vi "testDBMec.vi"() -> ()   [LabVIEW 2014]
panel:
  in  "FinMedicion":bool caption="Fin Medicion de Varillas?"
  in  "CreoEnDBTuplaTablaImagen":bool caption="Creo DB Tupla Imagen"
  in  "CreoEnDBTuplaTablaProductoAfterTuplaTablaReceta":bool caption="Insertar Tupla En DB Producto"
  in  "stop":bool
  in  "EstadoActual":string caption="Estado Actual de la Secuencia"
  in  "FinGuardadoMedicion":bool caption="Fin Del Guardado Medicion"
  in  "CreoDBTuplaVarilla":bool caption="Creo DB Tupla Varilla"
  in  "CreoMemorNuevoObjetoImagen":bool caption="Creo Memoria Nuevo Objeto Imagen"
  in  "CreoMemoriaNuevoObjetoRod":bool caption="Creo Memoria Nuevo Objeto Rod"
  in  "CreoEnDBTuplaTablaReceta":bool caption="Inserto Tupla Tabla Receta"
  in  "CreoObjetoRecetaNuevaODSteelGrade":bool caption="Creo Objeto Receta Nueva Para OD SG"
  in  "FinCreacionTuplasDB":bool caption="Fin Creacion Tuplas en DB Producto"
  in  "CreoTuplaEnDBProducto":bool caption="Insertar Tupla En DB Producto"
  in  "SeleccionarReceta":bool caption="Seleccionar Receta De Lista Mostrada"
  in  "MostrarListaRecetas":bool caption="Mostrar Lista de Recetas Existentes OD y SteelGrade"
  in  "VerificarExisteRecetaParaODYSteelGrade":bool caption="Verificar Existe Receta Para OD Y SteelGrade?"
  in  "CrearNuevoObjetoProducto":bool caption="Crear Nuevo Objeto Producto"
  in  "VerificarExisteProducto":bool caption="Verificar  Existe Producto?"
  in  "IngresarODSteelGradeLote":bool caption="Ingresar OD SteelGrade Lote"
  in  "RealizarMedicion":bool caption="Realizar Medicion"
  in  "NewProduct":bool caption="Nuevo Producto?"
  in  "Inicio":bool
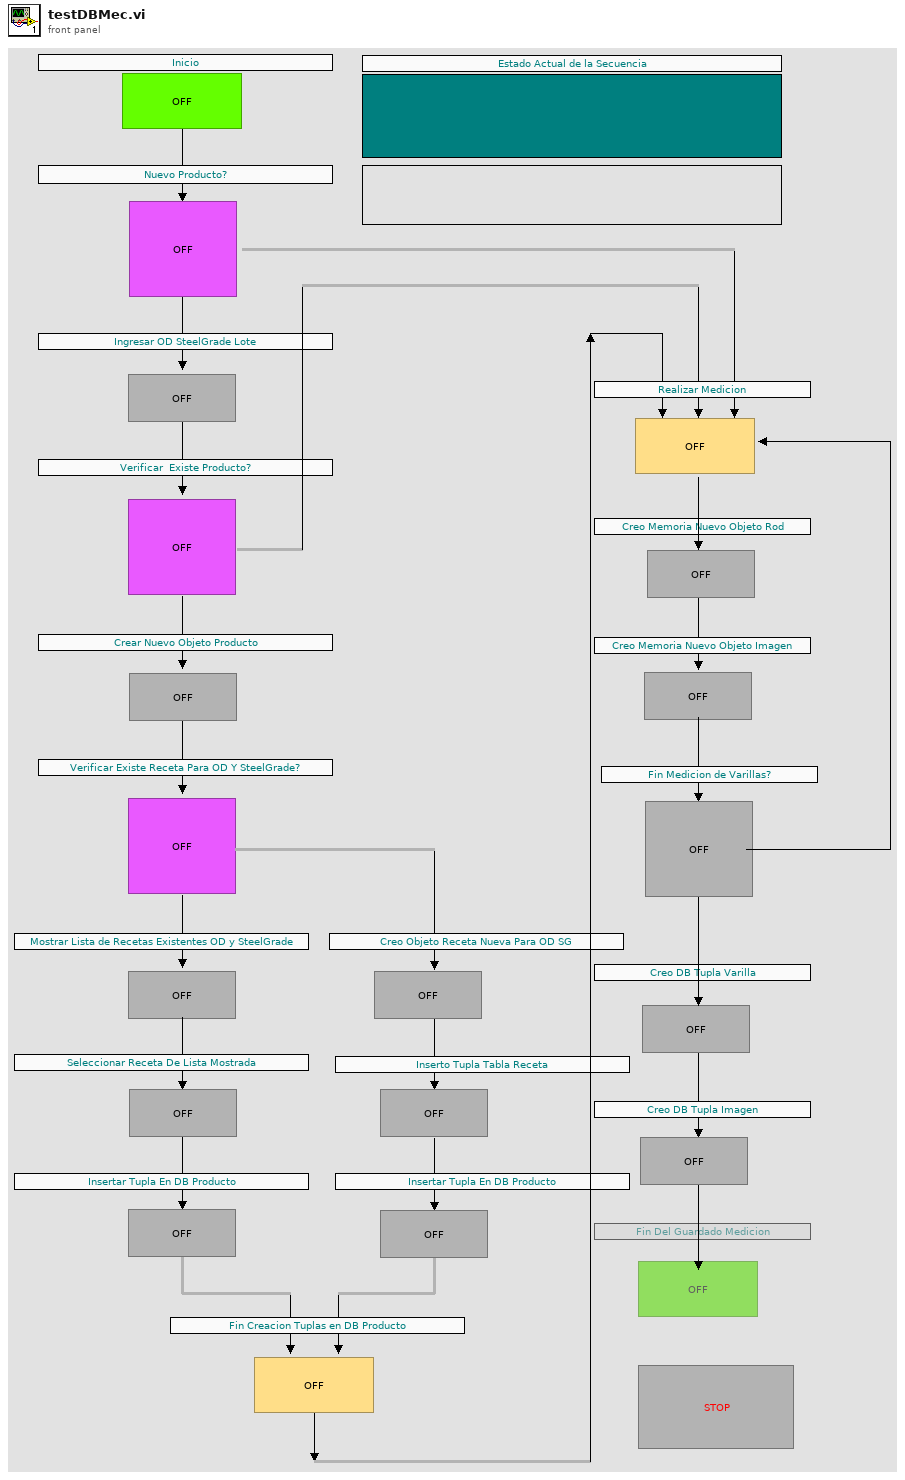
[diagram p1: front panel]
types:
  T1 = enum8{"Enabled", "Disabled", "Disabled and Grayed Out"}
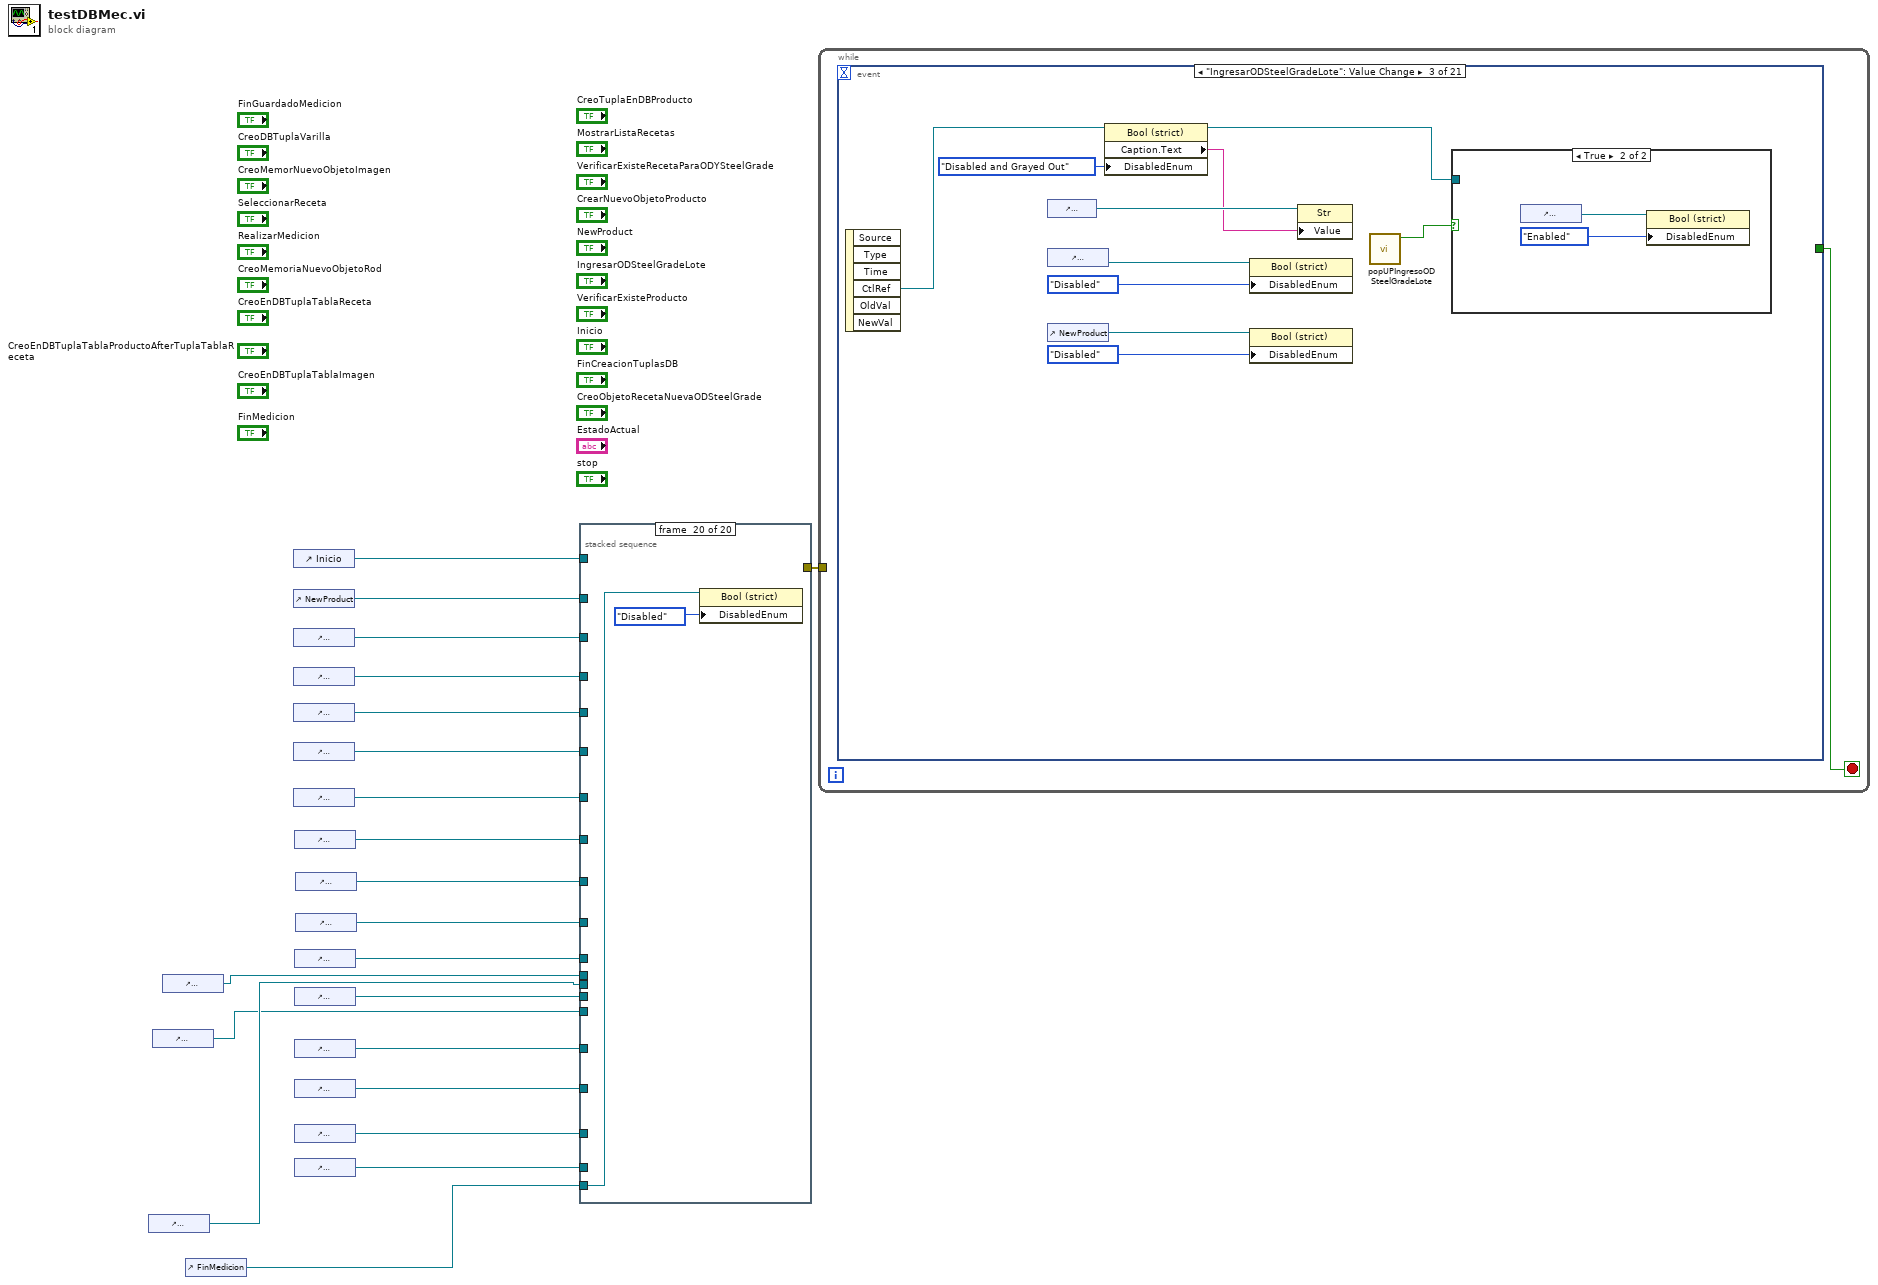
[diagram p0: block diagram]
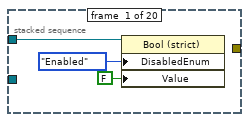
[diagram p2: hidden frame]
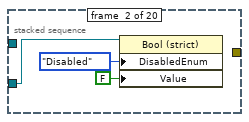
[diagram p3: hidden frame]
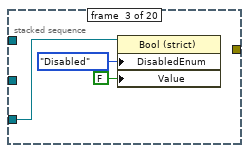
[diagram p4: hidden frame]
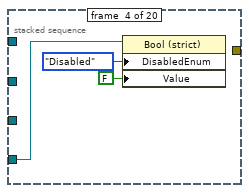
[diagram p5: hidden frame]
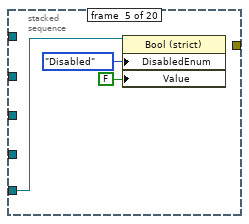
[diagram p6: hidden frame]
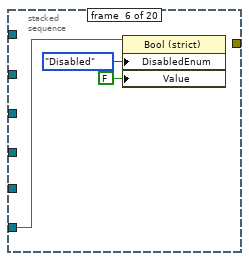
[diagram p7: hidden frame]
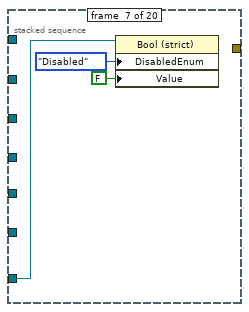
[diagram p8: hidden frame]
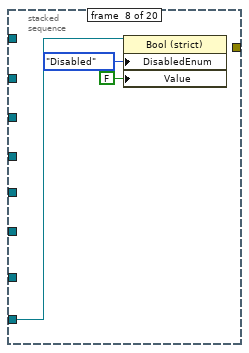
[diagram p9: hidden frame]
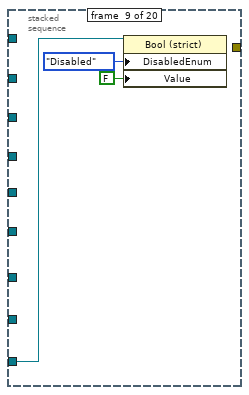
[diagram p10: hidden frame]
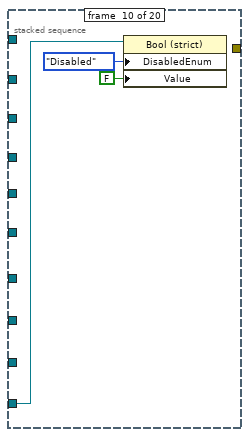
[diagram p11: hidden frame]
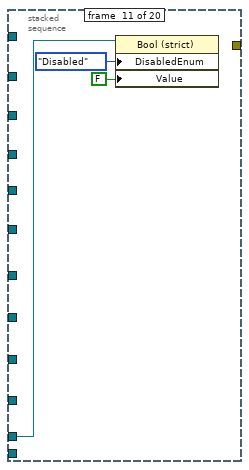
[diagram p12: hidden frame]
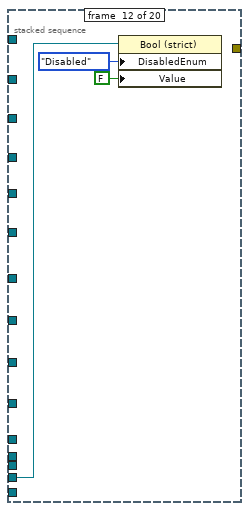
[diagram p13: hidden frame]
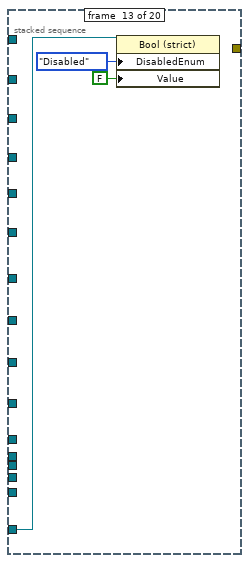
[diagram p14: hidden frame]
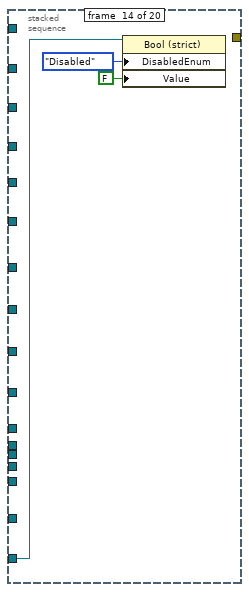
[diagram p15: hidden frame]
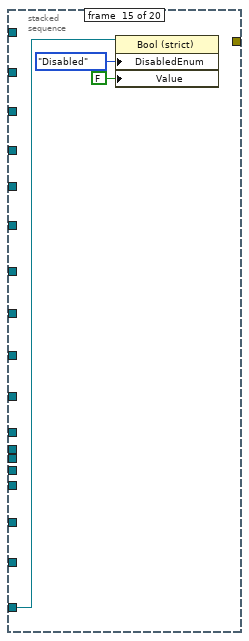
[diagram p16: hidden frame]
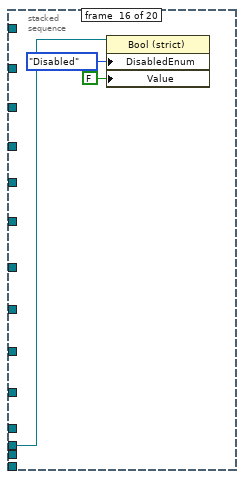
[diagram p17: hidden frame]
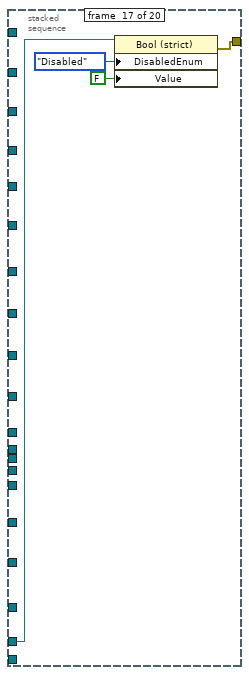
[diagram p18: hidden frame]
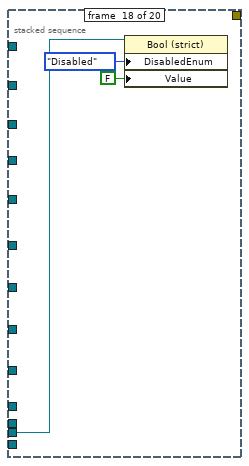
[diagram p19: hidden frame]
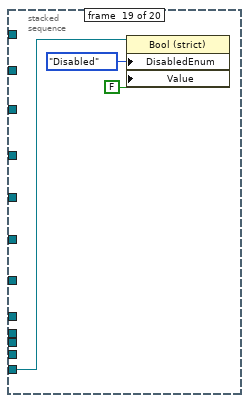
[diagram p20: hidden frame]
diagram:
  n1 = control-ref of="CreoEnDBTuplaTablaProductoAfterTuplaTablaReceta"() -> (w3:refnum<vi>)
  n2 = control-ref of="CreoEnDBTuplaTablaImagen"() -> (w2:refnum<vi>)
  n3 = control-ref of="FinCreacionTuplasDB"() -> (w4:refnum<vi>)
  n4 = control-ref of="FinMedicion"() -> (w1:refnum<vi>)
  n5 = control-ref of="Inicio"() -> (w21:refnum<vi>)
  n6 = control-ref of="NewProduct"() -> (w20:refnum<vi>)
  n7 = control-ref of="IngresarODSteelGradeLote"() -> (w19:refnum<vi>)
  n8 = control-ref of="VerificarExisteProducto"() -> (w18:refnum<vi>)
  n9 = control-ref of="CrearNuevoObjetoProducto"() -> (w17:refnum<vi>)
  n10 = control-ref of="VerificarExisteRecetaParaODYSteelGrade"() -> (w16:refnum<vi>)
  n11 = control-ref of="MostrarListaRecetas"() -> (w15:refnum<vi>)
  n12 = control-ref of="SeleccionarReceta"() -> (w14:refnum<vi>)
  n13 = control-ref of="CreoEnDBTuplaTablaReceta"() -> (w11:refnum<vi>)
  n14 = control-ref of="RealizarMedicion"() -> (w9:refnum<vi>)
  n15 = control-ref of="CreoMemoriaNuevoObjetoRod"() -> (w8:refnum<vi>)
  n16 = control-ref of="CreoMemorNuevoObjetoImagen"() -> (w7:refnum<vi>)
  n17 = control-ref of="CreoDBTuplaVarilla"() -> (w6:refnum<vi>)
  n18 = control-ref of="FinGuardadoMedicion"() -> (w5:refnum<vi>)
  n19 = control-ref of="CreoTuplaEnDBProducto"() -> (w13:refnum<vi>)
  n20 = control-ref of="CreoObjetoRecetaNuevaODSteelGrade"() -> (w12:refnum<vi>)
  n21 = stacked-sequence {
    tunnel: w21 -> [w24 _ _ _ _ _ _ _ _ _ _ _ _ _ _ _ _ _ _ _]
    tunnel: w20 -> [_ w27 _ _ _ _ _ _ _ _ _ _ _ _ _ _ _ _ _ _]
    tunnel: w19 -> [_ _ w30 _ _ _ _ _ _ _ _ _ _ _ _ _ _ _ _ _]
    tunnel: w18 -> [_ _ _ w33 _ _ _ _ _ _ _ _ _ _ _ _ _ _ _ _]
    tunnel: w17 -> [_ _ _ _ w36 _ _ _ _ _ _ _ _ _ _ _ _ _ _ _]
    tunnel: w16 -> [_ _ _ _ _ w39 _ _ _ _ _ _ _ _ _ _ _ _ _ _]
    tunnel: w15 -> [_ _ _ _ _ _ w42 _ _ _ _ _ _ _ _ _ _ _ _ _]
    tunnel: w14 -> [_ _ _ _ _ _ _ w45 _ _ _ _ _ _ _ _ _ _ _ _]
    tunnel: w13 -> [_ _ _ _ _ _ _ _ w48 _ _ _ _ _ _ _ _ _ _ _]
    tunnel: w12 -> [_ _ _ _ _ _ _ _ _ w51 _ _ _ _ _ _ _ _ _ _]
    tunnel: w11 -> [_ _ _ _ _ _ _ _ _ _ w54 _ _ _ _ _ _ _ _ _]
    tunnel: [_ _ _ _ _ _ _ _ _ _ _ _ _ _ _ _ w71 _ _ _] -> w10
    tunnel: w9 -> [_ _ _ _ _ _ _ _ _ _ _ w57 _ _ _ _ _ _ _ _]
    tunnel: w8 -> [_ _ _ _ _ _ _ _ _ _ _ _ w60 _ _ _ _ _ _ _]
    tunnel: w7 -> [_ _ _ _ _ _ _ _ _ _ _ _ _ w63 _ _ _ _ _ _]
    tunnel: w6 -> [_ _ _ _ _ _ _ _ _ _ _ _ _ _ w66 _ _ _ _ _]
    tunnel: w5 -> [_ _ _ _ _ _ _ _ _ _ _ _ _ _ _ _ w73 _ _ _]
    tunnel: w4 -> [_ _ _ _ _ _ _ _ _ _ _ _ _ _ _ w69 _ _ _ _]
    tunnel: w3 -> [_ _ _ _ _ _ _ _ _ _ _ _ _ _ _ _ _ w76 _ _]
    tunnel: w2 -> [_ _ _ _ _ _ _ _ _ _ _ _ _ _ _ _ _ _ w79 _]
    tunnel: w1 -> [_ _ _ _ _ _ _ _ _ _ _ _ _ _ _ _ _ _ _ w81]
    frame #0 {
      n22 = property class="Bool (strict)"(reference=w24, "DisabledEnum"=T1."Enabled" ("Disabled"), "Value"=FALSE) -> ()  [unwired: 1 in, 2 out]
    }
    frame #1 {
      n23 = property class="Bool (strict)"(reference=w27, "DisabledEnum"=T1."Disabled" ("Disabled"), "Value"=FALSE) -> ()  [unwired: 1 in, 2 out]
    }
    frame #2 {
      n24 = property class="Bool (strict)"(reference=w30, "DisabledEnum"=T1."Disabled" ("Disabled"), "Value"=FALSE) -> ()  [unwired: 1 in, 2 out]
    }
    frame #3 {
      n25 = property class="Bool (strict)"(reference=w33, "DisabledEnum"=T1."Disabled" ("Disabled"), "Value"=FALSE) -> ()  [unwired: 1 in, 2 out]
    }
    frame #4 {
      n26 = property class="Bool (strict)"(reference=w36, "DisabledEnum"=T1."Disabled" ("Disabled"), "Value"=FALSE) -> ()  [unwired: 1 in, 2 out]
    }
    frame #5 {
      n27 = property class="Bool (strict)"(reference=w39, "DisabledEnum"=T1."Disabled" ("Disabled"), "Value"=FALSE) -> ()  [unwired: 1 in, 2 out]
    }
    frame #6 {
      n28 = property class="Bool (strict)"(reference=w42, "DisabledEnum"=T1."Disabled" ("Disabled"), "Value"=FALSE) -> ()  [unwired: 1 in, 2 out]
    }
    frame #7 {
      n29 = property class="Bool (strict)"(reference=w45, "DisabledEnum"=T1."Disabled" ("Disabled"), "Value"=FALSE) -> ()  [unwired: 1 in, 2 out]
    }
    frame #8 {
      n30 = property class="Bool (strict)"(reference=w48, "DisabledEnum"=T1."Disabled" ("Disabled"), "Value"=FALSE) -> ()  [unwired: 1 in, 2 out]
    }
    frame #9 {
      n31 = property class="Bool (strict)"(reference=w51, "DisabledEnum"=T1."Disabled" ("Disabled"), "Value"=FALSE) -> ()  [unwired: 1 in, 2 out]
    }
    frame #10 {
      n32 = property class="Bool (strict)"(reference=w54, "DisabledEnum"=T1."Disabled" ("Disabled"), "Value"=FALSE) -> ()  [unwired: 1 in, 2 out]
    }
    frame #11 {
      n33 = property class="Bool (strict)"(reference=w57, "DisabledEnum"=T1."Disabled" ("Disabled"), "Value"=FALSE) -> ()  [unwired: 1 in, 2 out]
    }
    frame #12 {
      n34 = property class="Bool (strict)"(reference=w60, "DisabledEnum"=T1."Disabled" ("Disabled"), "Value"=FALSE) -> ()  [unwired: 1 in, 2 out]
    }
    frame #13 {
      n35 = property class="Bool (strict)"(reference=w63, "DisabledEnum"=T1."Disabled" ("Disabled"), "Value"=FALSE) -> ()  [unwired: 1 in, 2 out]
    }
    frame #14 {
      n36 = property class="Bool (strict)"(reference=w66, "DisabledEnum"=T1."Disabled" ("Disabled"), "Value"=FALSE) -> ()  [unwired: 1 in, 2 out]
    }
    frame #15 {
      n37 = property class="Bool (strict)"(reference=w69, "DisabledEnum"=T1."Disabled" ("Disabled"), "Value"=FALSE) -> ()  [unwired: 1 in, 2 out]
    }
    frame #16 {
      n38 = property class="Bool (strict)"(reference=w73, "DisabledEnum"=T1."Disabled" ("Disabled"), "Value"=FALSE) -> (error out=w71:errorcluster)  [unwired: 1 in, 1 out]
    }
    frame #17 {
      n39 = property class="Bool (strict)"(reference=w76, "DisabledEnum"=T1."Disabled" ("Disabled"), "Value"=FALSE) -> ()  [unwired: 1 in, 2 out]
    }
    frame #18 {
      n40 = property class="Bool (strict)"(reference=w79, "DisabledEnum"=T1."Disabled" ("Disabled"), "Value"=FALSE) -> ()  [unwired: 1 in, 2 out]
    }
    frame #19 {
      n41 = property class="Bool (strict)"(reference=w81, "DisabledEnum"=T1."Disabled" ("Disabled")) -> ()  [unwired: 1 in, 2 out]
    }
  }
  n42 = while {
    tunnel: w10 -> [_]
    stop <- w82 stop-if-true
    n43 = event shown="[2] \"IngresarODSteelGradeLote\": Value Change" {
      selector: _ -> [_ _ _ _ _ _ _ _ _ _ _ _ _ _ _ _ _ _ _ _ _]
      dyn-events: _ -> [_ _ _ _ _ _ _ _ _ _ _ _ _ _ _ _ _ _ _ _ _]
      timeout: _ -> [_ _ _ _ _ _ _ _ _ _ _ _ _ _ _ _ _ _ _ _ _]
      tunnel: [_ _ _ _ _ _ _ _ _ _ _ _ _ _ _ _ _ _ _ _ w355] -> w82
      event "Inicio": Value Change {
        n44 = event-data() -> ("CtlRef"=w88:refnum<vi>)  [unwired: 1 in, 5 out]
        n45 = control-ref of="EstadoActual"() -> (w87:refnum<vi>)
        n46 = control-ref of="NewProduct"() -> (w85:refnum<vi>)
        n47 = property class="Bool (strict)"(reference=w88, "DisabledEnum"=T1."Disabled and Grayed Out" ("Disabled")) -> ("Caption.Text"=w86:string)  [unwired: 1 in, 2 out]
        n48 = property class="Bool (strict)"(reference=w85, "DisabledEnum"=T1."Enabled" ("Disabled")) -> ()  [unwired: 1 in, 2 out]
        n49 = property class="Str"(reference=w87, "Value"=w86) -> ()  [unwired: 1 in, 2 out]
      }
      event "NewProduct": Value Change {
        n50 = event-data() -> ("CtlRef"=w95:refnum<vi>)  [unwired: 1 in, 5 out]
        n51 = control-ref of="EstadoActual"() -> (w94:refnum<vi>)
        n52 = control-ref of="Inicio"() -> (w92:refnum<vi>)
        n53 = property class="Bool (strict)"(reference=w95, "DisabledEnum"=T1."Disabled and Grayed Out" ("Disabled")) -> ("Caption.Text"=w93:string)  [unwired: 1 in, 2 out]
        n54 = property class="Bool (strict)"(reference=w92, "DisabledEnum"=T1."Disabled" ("Disabled")) -> ()  [unwired: 1 in, 2 out]
        n55 = property class="Str"(reference=w94, "Value"=w93) -> ()  [unwired: 1 in, 2 out]
        n56 = call "popUPSINO.vi"() -> ("estadoConsulta"=w89:bool)  [unwired: 11 in]
        n57 = case shown="False" w89 {
          frame False {
            n58 = control-ref of="RealizarMedicion"() -> (w96:refnum<vi>)
            n59 = property class="Bool (strict)"(reference=w96, "DisabledEnum"=T1."Enabled" ("Disabled")) -> ()  [unwired: 1 in, 2 out]
          }
          frame True {
            n60 = control-ref of="IngresarODSteelGradeLote"() -> (w99:refnum<vi>)
            n61 = property class="Bool (strict)"(reference=w99, "DisabledEnum"=T1."Enabled" ("Disabled")) -> ()  [unwired: 1 in, 2 out]
          }
        }
      }
      event "IngresarODSteelGradeLote": Value Change {
        n62 = event-data() -> ("CtlRef"=w109:refnum<vi>)  [unwired: 1 in, 5 out]
        n63 = control-ref of="EstadoActual"() -> (w108:refnum<vi>)
        n64 = control-ref of="RealizarMedicion"() -> (w104:refnum<vi>)
        n65 = control-ref of="NewProduct"() -> (w106:refnum<vi>)
        n66 = property class="Bool (strict)"(reference=w109, "DisabledEnum"=T1."Disabled and Grayed Out" ("Disabled")) -> (reference out=w101:refnum<vi>, "Caption.Text"=w107:string)  [unwired: 1 in, 1 out]
        n67 = property class="Bool (strict)"(reference=w104, "DisabledEnum"=T1."Disabled" ("Disabled")) -> ()  [unwired: 1 in, 2 out]
        n68 = property class="Bool (strict)"(reference=w106, "DisabledEnum"=T1."Disabled" ("Disabled")) -> ()  [unwired: 1 in, 2 out]
        n69 = property class="Str"(reference=w108, "Value"=w107) -> ()  [unwired: 1 in, 2 out]
        n70 = call "popUPIngresoODSteelGradeLote.vi"() -> ("Listo Ingresar OD SteelGrade Lote"=w100:bool)  [unwired: 10 in, 1 out]
        n71 = case shown="True" w100 {
          tunnel: w101 -> [_ _]
          frame False {
          }
          frame True {
            n72 = control-ref of="VerificarExisteProducto"() -> (w111:refnum<vi>)
            n73 = property class="Bool (strict)"(reference=w111, "DisabledEnum"=T1."Enabled" ("Disabled")) -> ()  [unwired: 1 in, 2 out]
          }
        }
      }
      event "VerificarExisteProducto": Value Change {
        n74 = event-data() -> ("CtlRef"=w118:refnum<vi>)  [unwired: 1 in, 5 out]
        n75 = control-ref of="EstadoActual"() -> (w117:refnum<vi>)
        n76 = control-ref of="IngresarODSteelGradeLote"() -> (w115:refnum<vi>)
        n77 = property class="Bool (strict)"(reference=w118, "DisabledEnum"=T1."Disabled and Grayed Out" ("Disabled")) -> ("Caption.Text"=w116:string)  [unwired: 1 in, 2 out]
        n78 = property class="Bool (strict)"(reference=w115, "DisabledEnum"=T1."Disabled" ("Disabled")) -> ()  [unwired: 1 in, 2 out]
        n79 = property class="Str"(reference=w117, "Value"=w116) -> ()  [unwired: 1 in, 2 out]
        n80 = call "popUPSINO.vi"() -> ("estadoConsulta"=w112:bool)  [unwired: 11 in]
        n81 = case shown="False" w112 {
          frame False {
            n82 = control-ref of="CrearNuevoObjetoProducto"() -> (w119:refnum<vi>)
            n83 = property class="Bool (strict)"(reference=w119, "DisabledEnum"=T1."Enabled" ("Disabled")) -> ()  [unwired: 1 in, 2 out]
          }
          frame True {
            n84 = control-ref of="RealizarMedicion"() -> (w121:refnum<vi>)
            n85 = property class="Bool (strict)"(reference=w121, "DisabledEnum"=T1."Enabled" ("Disabled")) -> ()  [unwired: 1 in, 2 out]
          }
        }
      }
      event "CrearNuevoObjetoProducto": Value Change {
        n86 = event-data() -> ("CtlRef"=w131:refnum<vi>)  [unwired: 1 in, 5 out]
        n87 = control-ref of="EstadoActual"() -> (w130:refnum<vi>)
        n88 = control-ref of="VerificarExisteProducto"() -> (w129:refnum<vi>)
        n89 = control-ref of="RealizarMedicion"() -> (w127:refnum<vi>)
        n90 = property class="Bool (strict)"(reference=w131, "DisabledEnum"=T1."Disabled and Grayed Out" ("Disabled")) -> ("Caption.Text"=w124:string)  [unwired: 1 in, 2 out]
        n91 = property class="Bool (strict)"(reference=w129, "DisabledEnum"=T1."Disabled" ("Disabled")) -> ()  [unwired: 1 in, 2 out]
        n92 = property class="Bool (strict)"(reference=w127, "DisabledEnum"=T1."Disabled" ("Disabled")) -> ()  [unwired: 1 in, 2 out]
        n93 = property class="Str"(reference=w130, "Value"=w124) -> ()  [unwired: 1 in, 2 out]
        n94 = call "popUPCrearNuevoObjetoProducto.vi"() -> ("Listo Ingresar objeto Producto"=w123:bool)  [unwired: 11 in]
        n95 = case shown="True" w123 {
          frame False {
          }
          frame True {
            n96 = control-ref of="VerificarExisteRecetaParaODYSteelGrade"() -> (w132:refnum<vi>)
            n97 = property class="Bool (strict)"(reference=w132, "DisabledEnum"=T1."Enabled" ("Disabled")) -> ()  [unwired: 1 in, 2 out]
          }
        }
      }
      event "VerificarExisteRecetaParaODYSteelGrade": Value Change {
        n98 = event-data() -> ("CtlRef"=w140:refnum<vi>)  [unwired: 1 in, 5 out]
        n99 = control-ref of="EstadoActual"() -> (w139:refnum<vi>)
        n100 = control-ref of="CrearNuevoObjetoProducto"() -> (w137:refnum<vi>)
        n101 = property class="Bool (strict)"(reference=w140, "DisabledEnum"=T1."Disabled and Grayed Out" ("Disabled")) -> ("Caption.Text"=w138:string)  [unwired: 1 in, 2 out]
        n102 = property class="Bool (strict)"(reference=w137, "DisabledEnum"=T1."Disabled" ("Disabled")) -> ()  [unwired: 1 in, 2 out]
        n103 = property class="Str"(reference=w139, "Value"=w138) -> ()  [unwired: 1 in, 2 out]
        n104 = call "popUPSINO.vi"() -> ("estadoConsulta"=w134:bool)  [unwired: 11 in]
        n105 = case shown="False" w134 {
          frame False {
            n106 = control-ref of="CreoObjetoRecetaNuevaODSteelGrade"() -> (w141:refnum<vi>)
            n107 = property class="Bool (strict)"(reference=w141, "DisabledEnum"=T1."Enabled" ("Disabled")) -> ()  [unwired: 1 in, 2 out]
          }
          frame True {
            n108 = control-ref of="MostrarListaRecetas"() -> (w143:refnum<vi>)
            n109 = property class="Bool (strict)"(reference=w143, "DisabledEnum"=T1."Enabled" ("Disabled")) -> ()  [unwired: 1 in, 2 out]
          }
        }
      }
      event "MostrarListaRecetas": Value Change {
        n110 = event-data() -> ("CtlRef"=w153:refnum<vi>)  [unwired: 1 in, 5 out]
        n111 = control-ref of="EstadoActual"() -> (w152:refnum<vi>)
        n112 = control-ref of="VerificarExisteRecetaParaODYSteelGrade"() -> (w150:refnum<vi>)
        n113 = control-ref of="CreoObjetoRecetaNuevaODSteelGrade"() -> (w148:refnum<vi>)
        n114 = property class="Bool (strict)"(reference=w153, "DisabledEnum"=T1."Disabled and Grayed Out" ("Disabled")) -> ("Caption.Text"=w151:string)  [unwired: 1 in, 2 out]
        n115 = property class="Bool (strict)"(reference=w150, "DisabledEnum"=T1."Disabled" ("Disabled")) -> ()  [unwired: 1 in, 2 out]
        n116 = property class="Bool (strict)"(reference=w148, "DisabledEnum"=T1."Disabled" ("Disabled")) -> ()  [unwired: 1 in, 2 out]
        n117 = property class="Str"(reference=w152, "Value"=w151) -> ()  [unwired: 1 in, 2 out]
        n118 = call "popUPConsultaListaRecetas.vi"() -> ("Listo ListarRecetas"=w145:bool)  [unwired: 11 in]
        n119 = case shown="True" w145 {
          frame False {
          }
          frame True {
            n120 = control-ref of="SeleccionarReceta"() -> (w154:refnum<vi>)
            n121 = property class="Bool (strict)"(reference=w154, "DisabledEnum"=T1."Enabled" ("Disabled")) -> ()  [unwired: 1 in, 2 out]
          }
        }
      }
      event "SeleccionarReceta": Value Change {
        n122 = event-data() -> ("CtlRef"=w164:refnum<vi>)  [unwired: 1 in, 5 out]
        n123 = control-ref of="EstadoActual"() -> (w163:refnum<vi>)
        n124 = control-ref of="MostrarListaRecetas"() -> (w161:refnum<vi>)
        n125 = property class="Bool (strict)"(reference=w164, "DisabledEnum"=T1."Disabled and Grayed Out" ("Disabled")) -> ("Caption.Text"=w162:string)  [unwired: 1 in, 2 out]
        n126 = property class="Bool (strict)"(reference=w161, "DisabledEnum"=T1."Disabled" ("Disabled")) -> ()  [unwired: 1 in, 2 out]
        n127 = property class="Str"(reference=w163, "Value"=w162) -> ()  [unwired: 1 in, 2 out]
        n128 = call "popUPSeleccionReceta.vi"() -> ("idReceta"=w156:string, "recetaSeleccionadaDeLaLista"=w157:string, "Listo SeleccionListaDeReceta"=w158:bool)  [unwired: 9 in]
        n129 = case shown="True" w158 {
          tunnel: w157 -> [_ _]
          tunnel: w156 -> [_ _]
          frame False {
          }
          frame True {
            n130 = control-ref of="CreoTuplaEnDBProducto"() -> (w165:refnum<vi>)
            n131 = property class="Bool (strict)"(reference=w165, "DisabledEnum"=T1."Enabled" ("Disabled")) -> ()  [unwired: 1 in, 2 out]
          }
        }
      }
      event "CreoTuplaEnDBProducto": Value Change {
        n132 = event-data() -> ("CtlRef"=w173:refnum<vi>)  [unwired: 1 in, 5 out]
        n133 = control-ref of="EstadoActual"() -> (w172:refnum<vi>)
        n134 = control-ref of="SeleccionarReceta"() -> (w170:refnum<vi>)
        n135 = property class="Bool (strict)"(reference=w173, "DisabledEnum"=T1."Disabled and Grayed Out" ("Disabled")) -> ("Caption.Text"=w171:string)  [unwired: 1 in, 2 out]
        n136 = property class="Bool (strict)"(reference=w170, "DisabledEnum"=T1."Disabled" ("Disabled")) -> ()  [unwired: 1 in, 2 out]
        n137 = property class="Str"(reference=w172, "Value"=w171) -> ()  [unwired: 1 in, 2 out]
        n138 = call "popUPInsertarTuplaEnDBProducto.vi"() -> ("ListoGuardarEnDB"=w167:bool)  [unwired: 11 in]
        n139 = case shown="True" w167 {
          frame False {
          }
          frame True {
            n140 = control-ref of="FinCreacionTuplasDB"() -> (w174:refnum<vi>)
            n141 = property class="Bool (strict)"(reference=w174, "DisabledEnum"=T1."Enabled" ("Disabled")) -> ()  [unwired: 1 in, 2 out]
          }
        }
      }
      event "CreoObjetoRecetaNuevaODSteelGrade": Value Change {
        n142 = event-data() -> ("CtlRef"=w184:refnum<vi>)  [unwired: 1 in, 5 out]
        n143 = control-ref of="EstadoActual"() -> (w183:refnum<vi>)
        n144 = control-ref of="VerificarExisteRecetaParaODYSteelGrade"() -> (w181:refnum<vi>)
        n145 = control-ref of="MostrarListaRecetas"() -> (w179:refnum<vi>)
        n146 = property class="Bool (strict)"(reference=w184, "DisabledEnum"=T1."Disabled and Grayed Out" ("Disabled")) -> ("Caption.Text"=w182:string)  [unwired: 1 in, 2 out]
        n147 = property class="Bool (strict)"(reference=w181, "DisabledEnum"=T1."Disabled" ("Disabled")) -> ()  [unwired: 1 in, 2 out]
        n148 = property class="Bool (strict)"(reference=w179, "DisabledEnum"=T1."Disabled" ("Disabled")) -> ()  [unwired: 1 in, 2 out]
        n149 = property class="Str"(reference=w183, "Value"=w182) -> ()  [unwired: 1 in, 2 out]
        n150 = call "popUPCrearNuevoObjetoReceta.vi"() -> ("Listo Ingresar OD SteelGrade Lote"=w176:bool)  [unwired: 10 in, 1 out]
        n151 = case shown="True" w176 {
          frame False {
          }
          frame True {
            n152 = control-ref of="CreoEnDBTuplaTablaReceta"() -> (w185:refnum<vi>)
            n153 = property class="Bool (strict)"(reference=w185, "DisabledEnum"=T1."Enabled" ("Disabled")) -> ()  [unwired: 1 in, 2 out]
          }
        }
      }
      event "CreoEnDBTuplaTablaReceta": Value Change {
        n154 = event-data() -> ("CtlRef"=w193:refnum<vi>)  [unwired: 1 in, 5 out]
        n155 = property class="Bool (strict)"(reference=w193, "DisabledEnum"=T1."Disabled and Grayed Out" ("Disabled")) -> ("Caption.Text"=w191:string)  [unwired: 1 in, 2 out]
        n156 = control-ref of="EstadoActual"() -> (w192:refnum<vi>)
        n157 = control-ref of="CreoObjetoRecetaNuevaODSteelGrade"() -> (w190:refnum<vi>)
        n158 = property class="Bool (strict)"(reference=w190, "DisabledEnum"=T1."Disabled" ("Disabled")) -> ()  [unwired: 1 in, 2 out]
        n159 = property class="Str"(reference=w192, "Value"=w191) -> ()  [unwired: 1 in, 2 out]
        n160 = call "popUPInsertarTuplaEnDBReceta.vi"() -> ("Listo Ingresar OD SteelGrade Lote"=w187:bool)  [unwired: 11 in]
        n161 = case shown="True" w187 {
          frame False {
          }
          frame True {
            n162 = control-ref of="CreoEnDBTuplaTablaProductoAfterTuplaTablaReceta"() -> (w194:refnum<vi>)
            n163 = property class="Bool (strict)"(reference=w194, "DisabledEnum"=T1."Enabled" ("Disabled")) -> ()  [unwired: 1 in, 2 out]
          }
        }
      }
      event "CreoEnDBTuplaTablaProductoAfterTuplaTablaReceta": Value Change {
        n164 = event-data() -> ("CtlRef"=w202:refnum<vi>)  [unwired: 1 in, 5 out]
        n165 = control-ref of="CreoEnDBTuplaTablaReceta"() -> (w198:refnum<vi>)
        n166 = property class="Bool (strict)"(reference=w202, "DisabledEnum"=T1."Disabled and Grayed Out" ("Disabled")) -> ("Caption.Text"=w199:string)  [unwired: 1 in, 2 out]
        n167 = control-ref of="EstadoActual"() -> (w200:refnum<vi>)
        n168 = property class="Bool (strict)"(reference=w198, "DisabledEnum"=T1."Disabled" ("Disabled")) -> ()  [unwired: 1 in, 2 out]
        n169 = property class="Str"(reference=w200, "Value"=w199) -> ()  [unwired: 1 in, 2 out]
        n170 = call "popUPInsertarTuplaEnDBProducto.vi"() -> ("ListoGuardarEnDB"=w196:bool)  [unwired: 11 in]
        n171 = case shown="True" w196 {
          frame False {
          }
          frame True {
            n172 = control-ref of="FinCreacionTuplasDB"() -> (w204:refnum<vi>)
            n173 = property class="Bool (strict)"(reference=w204, "DisabledEnum"=T1."Enabled" ("Disabled")) -> ()  [unwired: 1 in, 2 out]
          }
        }
      }
      event "FinCreacionTuplasDB": Value Change {
        n174 = event-data() -> ("CtlRef"=w214:refnum<vi>)  [unwired: 1 in, 5 out]
        n175 = control-ref of="EstadoActual"() -> (w213:refnum<vi>)
        n176 = control-ref of="CreoTuplaEnDBProducto"() -> (w211:refnum<vi>)
        n177 = control-ref of="RealizarMedicion"() -> (w208:refnum<vi>)
        n178 = control-ref of="CreoEnDBTuplaTablaProductoAfterTuplaTablaReceta"() -> (w205:refnum<vi>)
        n179 = property class="Bool (strict)"(reference=w214, "DisabledEnum"=T1."Disabled and Grayed Out" ("Disabled")) -> ("Caption.Text"=w212:string)  [unwired: 1 in, 2 out]
        n180 = property class="Bool (strict)"(reference=w211, "DisabledEnum"=T1."Disabled" ("Disabled")) -> ()  [unwired: 1 in, 2 out]
        n181 = property class="Bool (strict)"(reference=w205, "DisabledEnum"=T1."Disabled" ("Disabled")) -> ()  [unwired: 1 in, 2 out]
        n182 = property class="Bool (strict)"(reference=w208, "DisabledEnum"=T1."Enabled" ("Disabled")) -> ()  [unwired: 1 in, 2 out]
        n183 = property class="Str"(reference=w213, "Value"=w212) -> ()  [unwired: 1 in, 2 out]
      }
      event "RealizarMedicion": Value Change {
        n184 = event-data() -> ("CtlRef"=w230:refnum<vi>)  [unwired: 1 in, 5 out]
        n185 = control-ref of="EstadoActual"() -> (w229:refnum<vi>)
        n186 = control-ref of="FinCreacionTuplasDB"() -> (w227:refnum<vi>)
        n187 = control-ref of="VerificarExisteProducto"() -> (w225:refnum<vi>)
        n188 = control-ref of="NewProduct"() -> (w223:refnum<vi>)
        n189 = control-ref of="IngresarODSteelGradeLote"() -> (w219:refnum<vi>)
        n190 = control-ref of="CrearNuevoObjetoProducto"() -> (w217:refnum<vi>)
        n191 = control-ref of="CreoMemoriaNuevoObjetoRod"() -> (w221:refnum<vi>)
        n192 = property class="Bool (strict)"(reference=w230, "DisabledEnum"=T1."Disabled and Grayed Out" ("Disabled")) -> ("Caption.Text"=w228:string)  [unwired: 1 in, 2 out]
        n193 = property class="Bool (strict)"(reference=w227, "DisabledEnum"=T1."Disabled" ("Disabled")) -> ()  [unwired: 1 in, 2 out]
        n194 = property class="Bool (strict)"(reference=w225, "DisabledEnum"=T1."Disabled" ("Disabled")) -> ()  [unwired: 1 in, 2 out]
        n195 = property class="Bool (strict)"(reference=w223, "DisabledEnum"=T1."Disabled" ("Disabled")) -> ()  [unwired: 1 in, 2 out]
        n196 = property class="Bool (strict)"(reference=w219, "DisabledEnum"=T1."Disabled" ("Disabled")) -> ()  [unwired: 1 in, 2 out]
        n197 = property class="Bool (strict)"(reference=w217, "DisabledEnum"=T1."Disabled" ("Disabled")) -> ()  [unwired: 1 in, 2 out]
        n198 = property class="Bool (strict)"(reference=w221, "DisabledEnum"=T1."Enabled" ("Disabled")) -> ()  [unwired: 1 in, 2 out]
        n199 = property class="Str"(reference=w229, "Value"=w228) -> ()  [unwired: 1 in, 2 out]
      }
      event "CreoMemoriaNuevoObjetoRod": Value Change {
        n200 = event-data() -> ("CtlRef"=w237:refnum<vi>)  [unwired: 1 in, 5 out]
        n201 = control-ref of="EstadoActual"() -> (w236:refnum<vi>)
        n202 = control-ref of="RealizarMedicion"() -> (w234:refnum<vi>)
        n203 = property class="Bool (strict)"(reference=w237, "DisabledEnum"=T1."Disabled and Grayed Out" ("Disabled")) -> ("Caption.Text"=w235:string)  [unwired: 1 in, 2 out]
        n204 = property class="Bool (strict)"(reference=w234, "DisabledEnum"=T1."Disabled" ("Disabled")) -> ()  [unwired: 1 in, 2 out]
        n205 = property class="Str"(reference=w236, "Value"=w235) -> ()  [unwired: 1 in, 2 out]
        n206 = call "popUPCrearNuevoObjetoRod.vi"() -> ("Listo Ingresar OD SteelGrade Lote"=w231:bool)  [unwired: 10 in, 1 out]
        n207 = case shown="True" w231 {
          frame False {
          }
          frame True {
            n208 = control-ref of="CreoMemorNuevoObjetoImagen"() -> (w238:refnum<vi>)
            n209 = property class="Bool (strict)"(reference=w238, "DisabledEnum"=T1."Enabled" ("Disabled")) -> ()  [unwired: 1 in, 2 out]
          }
        }
      }
      event "CreoMemorNuevoObjetoImagen": Value Change {
        n210 = event-data() -> ("CtlRef"=w246:refnum<vi>)  [unwired: 1 in, 5 out]
        n211 = control-ref of="EstadoActual"() -> (w245:refnum<vi>)
        n212 = control-ref of="CreoMemoriaNuevoObjetoRod"() -> (w243:refnum<vi>)
        n213 = property class="Bool (strict)"(reference=w246, "DisabledEnum"=T1."Disabled and Grayed Out" ("Disabled")) -> ("Caption.Text"=w244:string)  [unwired: 1 in, 2 out]
        n214 = property class="Bool (strict)"(reference=w243, "DisabledEnum"=T1."Disabled" ("Disabled")) -> ()  [unwired: 1 in, 2 out]
        n215 = property class="Str"(reference=w245, "Value"=w244) -> ()  [unwired: 1 in, 2 out]
        n216 = call "popUPCrearNuevoObjetoImagen.vi"() -> ("Listo Ingresar Datos Imagen"=w240:bool)  [unwired: 10 in, 1 out]
        n217 = case shown="True" w240 {
          frame False {
          }
          frame True {
            n218 = control-ref of="FinMedicion"() -> (w247:refnum<vi>)
            n219 = property class="Bool (strict)"(reference=w247, "DisabledEnum"=T1."Enabled" ("Disabled")) -> ()  [unwired: 1 in, 2 out]
          }
        }
      }
      event "FinMedicion": Value Change {
        n220 = event-data() -> ("CtlRef"=w256:refnum<vi>)  [unwired: 1 in, 5 out]
        n221 = control-ref of="CreoMemorNuevoObjetoImagen"() -> (w252:refnum<vi>)
        n222 = property class="Bool (strict)"(reference=w256, "DisabledEnum"=T1."Disabled and Grayed Out" ("Disabled")) -> (reference out=w249:refnum<vi>, "Caption.Text"=w253:string)  [unwired: 1 in, 1 out]
        n223 = control-ref of="EstadoActual"() -> (w254:refnum<vi>)
        n224 = property class="Bool (strict)"(reference=w252, "DisabledEnum"=T1."Disabled" ("Disabled")) -> ()  [unwired: 1 in, 2 out]
        n225 = property class="Str"(reference=w254, "Value"=w253) -> ()  [unwired: 1 in, 2 out]
        n226 = call "popUPSINO.vi"() -> ("estadoConsulta"=w250:bool)  [unwired: 11 in]
        n227 = case shown="False" w250 {
          tunnel: w249 -> [w259 _]
          frame False {
            n228 = control-ref of="RealizarMedicion"() -> (w266:refnum<vi>)
            n229 = control-ref of="CreoMemoriaNuevoObjetoRod"() -> (w264:refnum<vi>)
            n230 = control-ref of="CreoMemorNuevoObjetoImagen"() -> (w262:refnum<vi>)
            n231 = property class="Bool (strict)"(reference=w259, "Value"=FALSE, "DisabledEnum"=T1."Disabled" ("Disabled")) -> ()  [unwired: 1 in, 2 out]
            n232 = property class="Bool (strict)"(reference=w262, "Value"=FALSE) -> ()  [unwired: 1 in, 2 out]
            n233 = property class="Bool (strict)"(reference=w266, "Value"=FALSE, "DisabledEnum"=T1."Enabled" ("Disabled")) -> ()  [unwired: 1 in, 2 out]
            n234 = property class="Bool (strict)"(reference=w264, "Value"=FALSE) -> ()  [unwired: 1 in, 2 out]
          }
          frame True {
            n235 = control-ref of="CreoDBTuplaVarilla"() -> (w268:refnum<vi>)
            n236 = property class="Bool (strict)"(reference=w268, "DisabledEnum"=T1."Enabled" ("Disabled")) -> ()  [unwired: 1 in, 2 out]
          }
        }
      }
      event "CreoDBTuplaVarilla": Value Change {
        n237 = event-data() -> ("CtlRef"=w275:refnum<vi>)  [unwired: 1 in, 5 out]
        n238 = control-ref of="FinMedicion"() -> (w269:refnum<vi>)
        n239 = control-ref of="EstadoActual"() -> (w274:refnum<vi>)
        n240 = property class="Bool (strict)"(reference=w275, "DisabledEnum"=T1."Disabled and Grayed Out" ("Disabled")) -> ("Caption.Text"=w273:string)  [unwired: 1 in, 2 out]
        n241 = property class="Bool (strict)"(reference=w269, "DisabledEnum"=T1."Disabled" ("Disabled")) -> ()  [unwired: 1 in, 2 out]
        n242 = property class="Str"(reference=w274, "Value"=w273) -> ()  [unwired: 1 in, 2 out]
        n243 = call "popUPInsertarTuplaEnDBVarilla.vi"() -> ("ListoGuardarEnDB"=w270:bool)  [unwired: 11 in]
        n244 = case shown="True" w270 {
          frame False {
          }
          frame True {
            n245 = control-ref of="CreoEnDBTuplaTablaImagen"() -> (w276:refnum<vi>)
            n246 = property class="Bool (strict)"(reference=w276, "DisabledEnum"=T1."Enabled" ("Disabled")) -> ()  [unwired: 1 in, 2 out]
          }
        }
      }
      event "CreoEnDBTuplaTablaImagen": Value Change {
        n247 = event-data() -> ("CtlRef"=w284:refnum<vi>)  [unwired: 1 in, 5 out]
        n248 = property class="Bool (strict)"(reference=w284, "DisabledEnum"=T1."Disabled and Grayed Out" ("Disabled")) -> ("Caption.Text"=w281:string)  [unwired: 1 in, 2 out]
        n249 = control-ref of="CreoDBTuplaVarilla"() -> (w280:refnum<vi>)
        n250 = control-ref of="EstadoActual"() -> (w282:refnum<vi>)
        n251 = property class="Bool (strict)"(reference=w280, "DisabledEnum"=T1."Disabled" ("Disabled")) -> ()  [unwired: 1 in, 2 out]
        n252 = property class="Str"(reference=w282, "Value"=w281) -> ()  [unwired: 1 in, 2 out]
        n253 = call "popUPInsertarTuplaEnDBImagen.vi"() -> ("ListoGuardarEnDB"=w278:bool)  [unwired: 11 in]
        n254 = case shown="True" w278 {
          frame False {
          }
          frame True {
            n255 = control-ref of="FinGuardadoMedicion"() -> (w286:refnum<vi>)
            n256 = property class="Bool (strict)"(reference=w286, "DisabledEnum"=T1."Enabled" ("Disabled")) -> ()  [unwired: 1 in, 2 out]
          }
        }
      }
      event "FinGuardadoMedicion": Value Change {
        n257 = event-data() -> ("CtlRef"=w354:refnum<vi>)  [unwired: 1 in, 5 out]
        n258 = control-ref of="VerificarExisteProducto"() -> (w302:refnum<vi>)
        n259 = control-ref of="VerificarExisteProducto"() -> (w299:refnum<vi>)
        n260 = control-ref of="IngresarODSteelGradeLote"() -> (w296:refnum<vi>)
        n261 = control-ref of="NewProduct"() -> (w293:refnum<vi>)
        n262 = control-ref of="Inicio"() -> (w290:refnum<vi>)
        n263 = property class="Bool (strict)"(reference=w354, "DisabledEnum"=T1."Disabled and Grayed Out" ("Disabled"), "Value"=FALSE) -> ("Caption.Text"=w352:string)  [unwired: 1 in, 2 out]
        n264 = control-ref of="EstadoActual"() -> (w353:refnum<vi>)
        n265 = property class="Bool (strict)"(reference=w302, "DisabledEnum"=T1."Disabled" ("Disabled"), "Value"=FALSE) -> ()  [unwired: 1 in, 2 out]
        n266 = property class="Bool (strict)"(reference=w299, "DisabledEnum"=T1."Disabled" ("Disabled"), "Value"=FALSE) -> ()  [unwired: 1 in, 2 out]
        n267 = property class="Bool (strict)"(reference=w296, "DisabledEnum"=T1."Disabled" ("Disabled"), "Value"=FALSE) -> ()  [unwired: 1 in, 2 out]
        n268 = property class="Bool (strict)"(reference=w293, "DisabledEnum"=T1."Disabled" ("Disabled"), "Value"=FALSE) -> ()  [unwired: 1 in, 2 out]
        n269 = property class="Bool (strict)"(reference=w290, "DisabledEnum"=T1."Enabled" ("Disabled"), "Value"=FALSE) -> ()  [unwired: 1 in, 2 out]
        n270 = property class="Str"(reference=w353, "Value"=w352) -> ()  [unwired: 1 in, 2 out]
        n271 = control-ref of="CreoEnDBTuplaTablaImagen"() -> (w350:refnum<vi>)
        n272 = control-ref of="CreoEnDBTuplaTablaImagen"() -> (w347:refnum<vi>)
        n273 = control-ref of="CreoDBTuplaVarilla"() -> (w344:refnum<vi>)
        n274 = control-ref of="FinMedicion"() -> (w341:refnum<vi>)
        n275 = control-ref of="CreoMemorNuevoObjetoImagen"() -> (w338:refnum<vi>)
        n276 = control-ref of="CreoMemoriaNuevoObjetoRod"() -> (w335:refnum<vi>)
        n277 = control-ref of="RealizarMedicion"() -> (w332:refnum<vi>)
        n278 = control-ref of="FinCreacionTuplasDB"() -> (w329:refnum<vi>)
        n279 = property class="Bool (strict)"(reference=w350, "DisabledEnum"=T1."Disabled" ("Disabled"), "Value"=FALSE) -> ()  [unwired: 1 in, 2 out]
        n280 = property class="Bool (strict)"(reference=w347, "DisabledEnum"=T1."Disabled" ("Disabled"), "Value"=FALSE) -> ()  [unwired: 1 in, 2 out]
        n281 = property class="Bool (strict)"(reference=w344, "DisabledEnum"=T1."Disabled" ("Disabled"), "Value"=FALSE) -> ()  [unwired: 1 in, 2 out]
        n282 = property class="Bool (strict)"(reference=w341, "DisabledEnum"=T1."Disabled" ("Disabled"), "Value"=FALSE) -> ()  [unwired: 1 in, 2 out]
        n283 = property class="Bool (strict)"(reference=w338, "DisabledEnum"=T1."Disabled" ("Disabled"), "Value"=FALSE) -> ()  [unwired: 1 in, 2 out]
        n284 = property class="Bool (strict)"(reference=w335, "DisabledEnum"=T1."Disabled" ("Disabled"), "Value"=FALSE) -> ()  [unwired: 1 in, 2 out]
        n285 = property class="Bool (strict)"(reference=w332, "DisabledEnum"=T1."Disabled" ("Disabled"), "Value"=FALSE) -> ()  [unwired: 1 in, 2 out]
        n286 = property class="Bool (strict)"(reference=w329, "DisabledEnum"=T1."Disabled" ("Disabled"), "Value"=FALSE) -> ()  [unwired: 1 in, 2 out]
        n287 = control-ref of="CreoTuplaEnDBProducto"() -> (w326:refnum<vi>)
        n288 = control-ref of="CreoEnDBTuplaTablaProductoAfterTuplaTablaReceta"() -> (w323:refnum<vi>)
        n289 = control-ref of="SeleccionarReceta"() -> (w320:refnum<vi>)
        n290 = control-ref of="CreoEnDBTuplaTablaReceta"() -> (w317:refnum<vi>)
        n291 = control-ref of="MostrarListaRecetas"() -> (w314:refnum<vi>)
        n292 = control-ref of="CreoObjetoRecetaNuevaODSteelGrade"() -> (w311:refnum<vi>)
        n293 = control-ref of="VerificarExisteRecetaParaODYSteelGrade"() -> (w308:refnum<vi>)
        n294 = control-ref of="CrearNuevoObjetoProducto"() -> (w305:refnum<vi>)
        n295 = property class="Bool (strict)"(reference=w326, "DisabledEnum"=T1."Disabled" ("Disabled"), "Value"=FALSE) -> ()  [unwired: 1 in, 2 out]
        n296 = property class="Bool (strict)"(reference=w323, "DisabledEnum"=T1."Disabled" ("Disabled"), "Value"=FALSE) -> ()  [unwired: 1 in, 2 out]
        n297 = property class="Bool (strict)"(reference=w320, "DisabledEnum"=T1."Disabled" ("Disabled"), "Value"=FALSE) -> ()  [unwired: 1 in, 2 out]
        n298 = property class="Bool (strict)"(reference=w317, "DisabledEnum"=T1."Disabled" ("Disabled"), "Value"=FALSE) -> ()  [unwired: 1 in, 2 out]
        n299 = property class="Bool (strict)"(reference=w314, "DisabledEnum"=T1."Disabled" ("Disabled"), "Value"=FALSE) -> ()  [unwired: 1 in, 2 out]
        n300 = property class="Bool (strict)"(reference=w311, "DisabledEnum"=T1."Disabled" ("Disabled"), "Value"=FALSE) -> ()  [unwired: 1 in, 2 out]
        n301 = property class="Bool (strict)"(reference=w308, "DisabledEnum"=T1."Disabled" ("Disabled"), "Value"=FALSE) -> ()  [unwired: 1 in, 2 out]
        n302 = property class="Bool (strict)"(reference=w305, "Value"=FALSE, "DisabledEnum"=T1."Disabled" ("Disabled")) -> ()  [unwired: 1 in, 2 out]
      }
      event "stop": Value Change {
        n303 = event-data() -> ("CtlRef"=w356:refnum<vi>)  [unwired: 1 in, 5 out]
        n304 = property class="Bool (strict)"(reference=w356) -> ("Value"=w355:bool)  [unwired: 1 in, 2 out]
      }
    }
  }
